vi "Piano PWM AO.vi"() -> ()   [LabVIEW 2024, in "CTI-Scratchpad.lvlib"]
uses:
  CTI/Identity.ctl
  CTI/GPIO Number.ctl
  CTI/Session/Session.lvclass
  CTI-Scratchpad.lvlib
  CTI/VisaComms/VisaComms.lvclass
  CTI/CTI.lvlib
panel:
  out "Identity":T1
  in  "GroveConnector":enum16{"A0", "A1", "A2"}(ring)
  out "error out":errorcluster
  in  "Duty Cycle":dbl(slide)=0.09183673469387754 scale=0.0..1.0
  in  "D5#":bool
  in  "E5":bool
  in  "C5#":bool
  in  "D5":bool
  in  "A4#":bool
  in  "G4#":bool
  in  "F4#":bool
  in  "D4#":bool
  in  "C4#":bool
  in  "VISA resource":refnum<visa-resource-name>="ASRL5::INSTR"
  in  "stop":bool
  in  "C5":bool
  in  "B4":bool
  in  "A4":bool
  in  "G4":bool
  in  "F4":bool
  in  "E4":bool
  in  "D4":bool
  in  "C4":bool
  # "https://wiki.seeedstudio.com/Grove-Passive-Buzzer/"
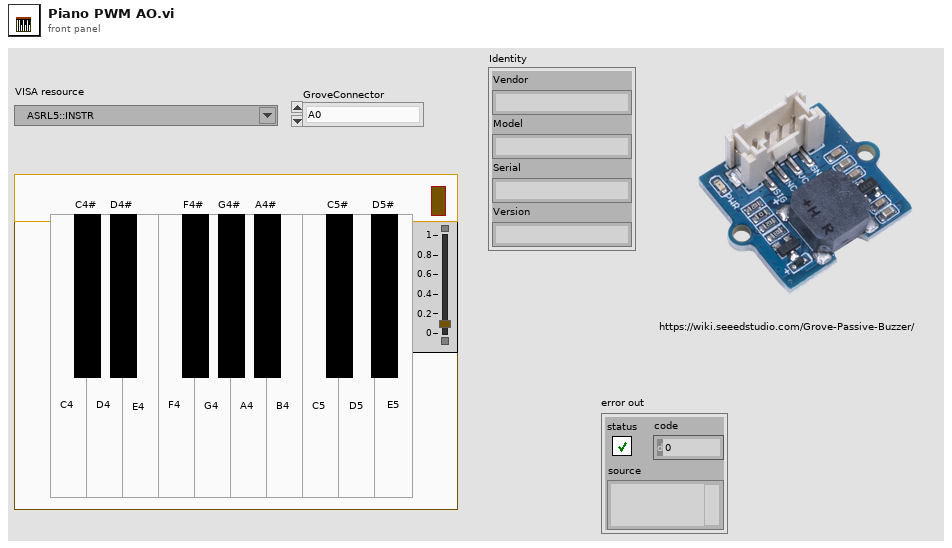
[diagram p1: front panel]
types:
  T1 = typedef "CTI.lvlib/Identity.ctl" = cluster{"Vendor":string, "Model":string, "Serial":string, "Version":string}
  T2 = typedef "CTI.lvlib/GPIO Number.ctl" = i8
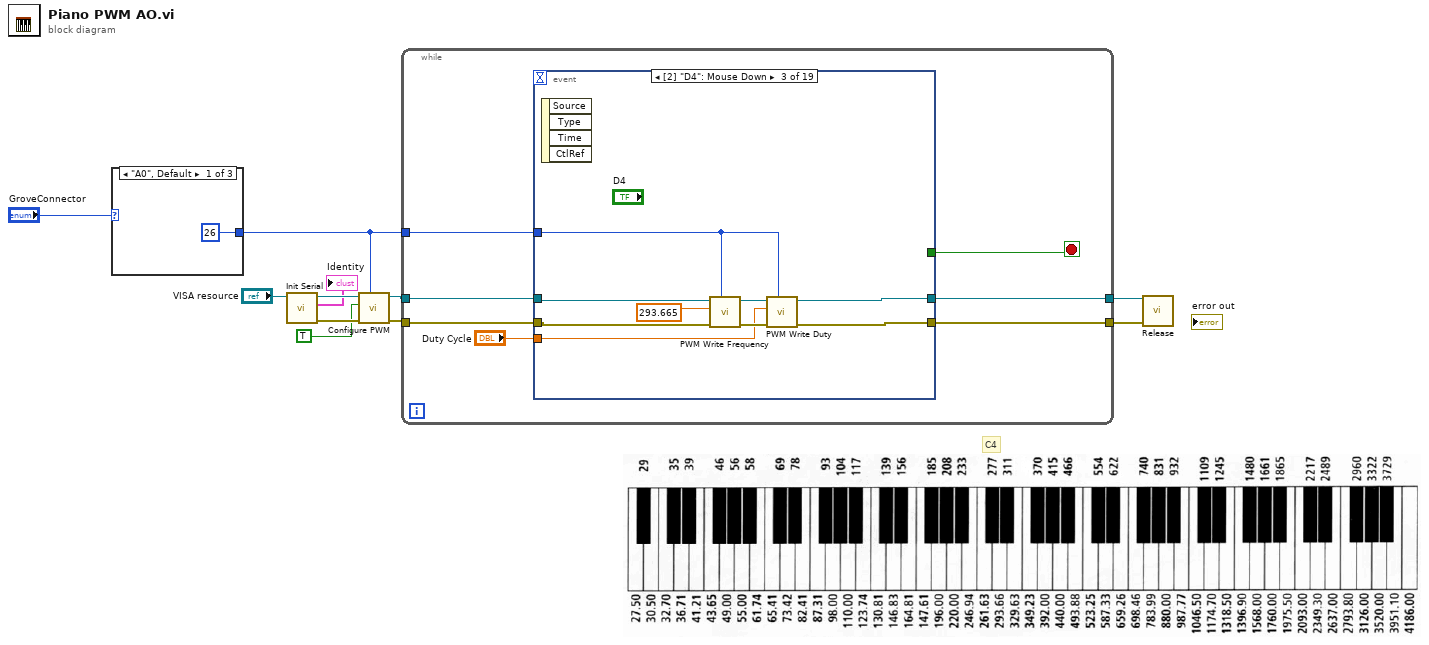
[diagram p0: block diagram]
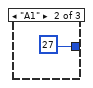
[diagram p2: hidden frame]
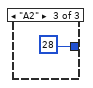
[diagram p3: hidden frame]
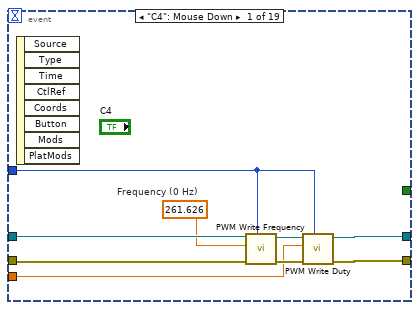
[diagram p4: hidden frame]
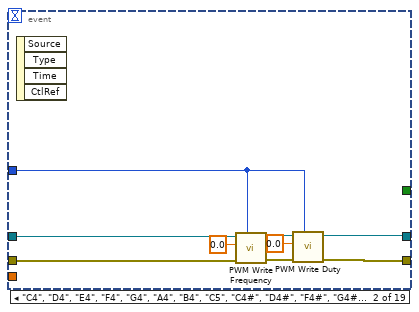
[diagram p5: hidden frame]
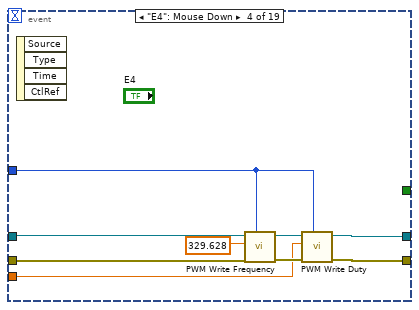
[diagram p6: hidden frame]
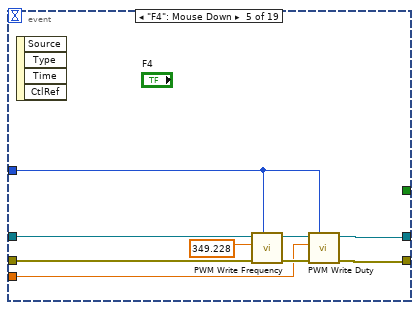
[diagram p7: hidden frame]
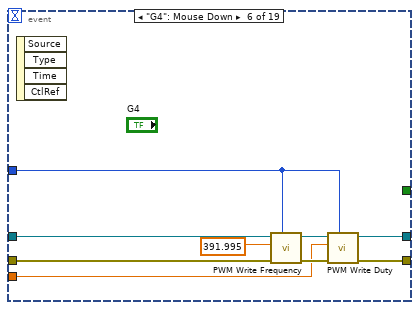
[diagram p8: hidden frame]
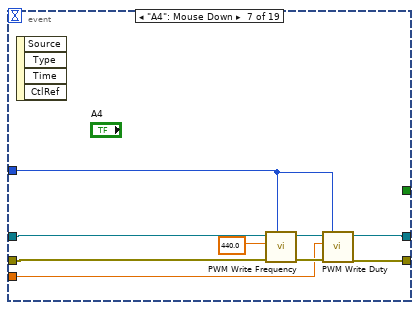
[diagram p9: hidden frame]
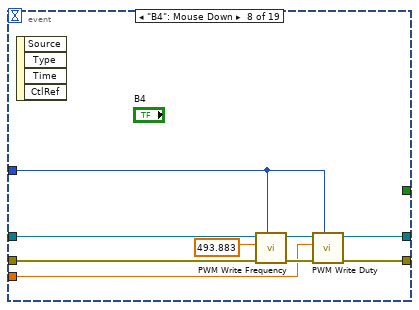
[diagram p10: hidden frame]
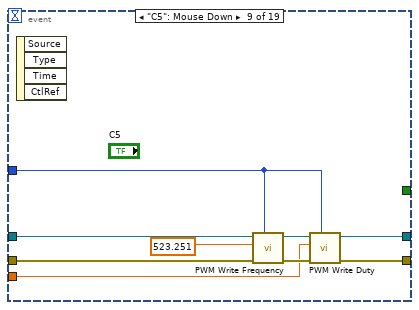
[diagram p11: hidden frame]
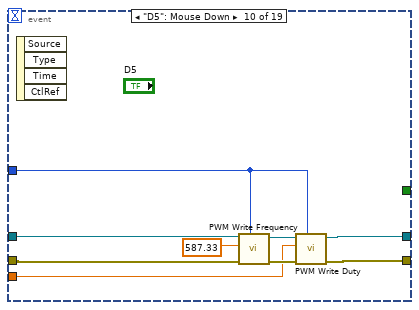
[diagram p12: hidden frame]
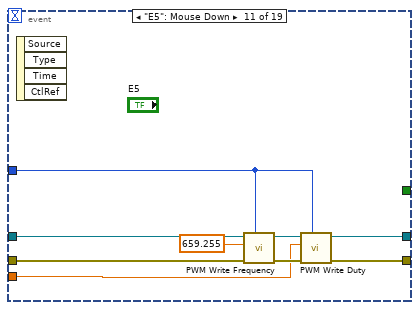
[diagram p13: hidden frame]
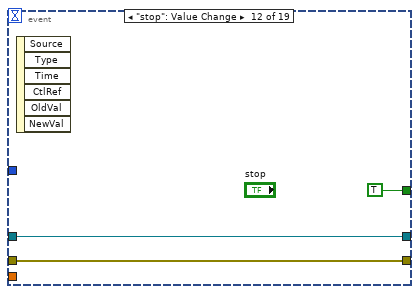
[diagram p14: hidden frame]
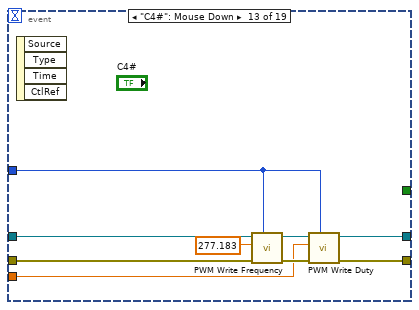
[diagram p15: hidden frame]
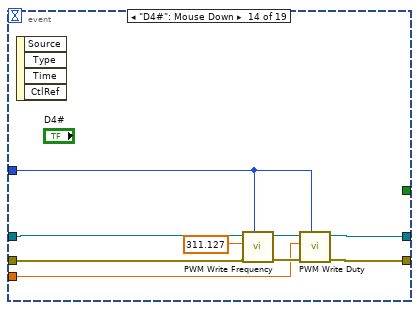
[diagram p16: hidden frame]
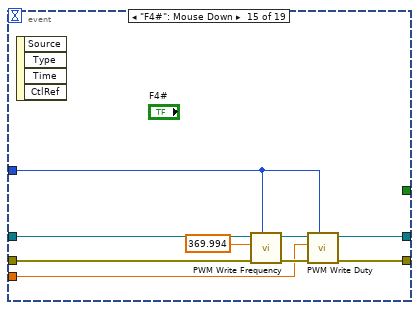
[diagram p17: hidden frame]
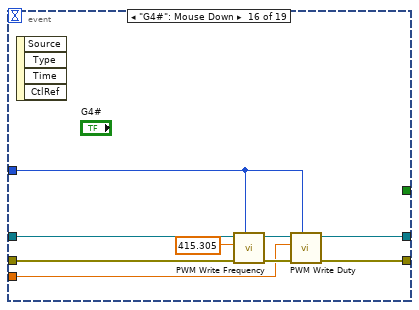
[diagram p18: hidden frame]
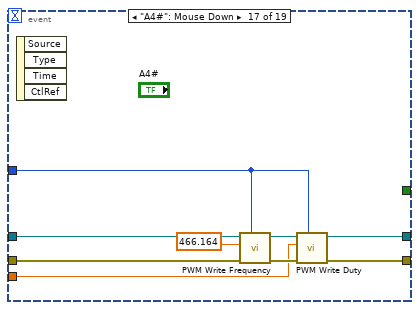
[diagram p19: hidden frame]
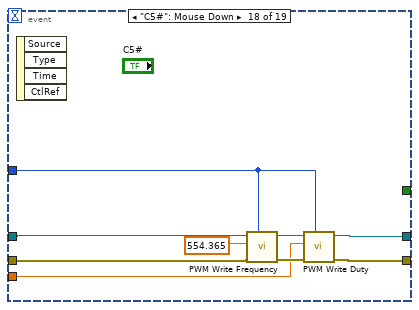
[diagram p20: hidden frame]
diagram:
  # "C4"
  n1 = case shown="\"A0\", Default" "GroveConnector" {
    tunnel: [T2 26 ("GPIO #") T2 27 ("GPIO #") T2 28 ("GPIO #")] -> w3
    frame "A0", Default {
    }
    frame "A1" {
    }
    frame "A2" {
    }
  }
  n2 = call "Init Serial.vi"("VISA resource name in"="VISA resource") -> ("error out"=w9:errorcluster, "Identity"=→"Identity":T1, "Session"=w10:refnum<class "Session.lvclass">)  [unwired: 8 in]
  n3 = call "Configure PWM.vi"("GPIO #"=w3, "error in (no error)"=w9, "Enable (F)"=TRUE, "Session in"=w10) -> ("error out"=w6:errorcluster, "Session out"=w5:refnum<class "Session.lvclass">)  [unwired: 6 in]
  n4 = while {
    tunnel: w5 -> [w20]
    tunnel: w6 -> [w19]
    tunnel: [w16] -> w4
    tunnel: [w17] -> w2
    tunnel: w3 -> [w15]
    stop <- w18 stop-if-true
    n5 = event shown="[2] \"D4\": Mouse Down" {
      selector: _ -> [_ _ _ _ _ _ _ _ _ _ _ _ _ _ _ _ _ _ _]
      dyn-events: _ -> [_ _ _ _ _ _ _ _ _ _ _ _ _ _ _ _ _ _ _]
      timeout: _ -> [_ _ _ _ _ _ _ _ _ _ _ _ _ _ _ _ _ _ _]
      tunnel: "Duty Cycle" -> [w23 _ w44 w53 w61 w69 w80 w85 w95 w103 w113 _ w125 w134 w142 w151 w160 w169 w178]
      tunnel: w20 -> [w25 w37 w47 w55 w64 w71 w78 w90 w97 w106 w116 w122 w127 w136 w145 w155 w163 w173 w181]
      tunnel: w19 -> [w26 w36 w45 w54 w63 w68 w79 w91 w98 w107 w117 w121 w128 w135 w146 w154 w164 w172 w182]
      tunnel: [w27 w35 w41 w49 w59 w72 w81 w87 w94 w108 w118 w121 w129 w138 w147 w156 w165 w174 w183] -> w16
      tunnel: [w28 w34 w42 w50 w60 w73 w82 w88 w100 w109 w114 w122 w130 w139 w148 w157 w166 w175 w184] -> w17
      tunnel: [_ _ _ _ _ _ _ _ _ _ _ TRUE _ _ _ _ _ _ _] -> w18
      tunnel: w15 -> [w22 w33 w40 w51 w58 w67 w76 w89 w99 w104 w115 _ w126 w137 w144 w153 w162 w171 w180]
      event "C4": Mouse Down {
        w24 = 261.626  # Frequency (0 Hz)
        n6 = event-data() -> ()  [unwired: 1 in, 8 out]
        n7 = call "PWM Write Frequency.vi"("GPIO #"=w22, "error in (no error)"=w26, "Frequency Hz"=w24, "Session in"=w25) -> ("error out"=w30:errorcluster, "Session out"=w29:refnum<class "Session.lvclass">)  [unwired: 6 in]
        n8 = call "PWM Write Duty.vi"("GPIO #"=w22, "error in (no error)"=w30, "Duty % (0-1)"=w23, "Session in"=w29) -> ("error out"=w27:errorcluster, "Session out"=w28:refnum<class "Session.lvclass">)  [unwired: 6 in]
      }
      event "C4", "D4", "E4", "F4", "G4", "A4", "B4", "C5", "C4#", "D4#", "F4#", "G4#", "A4#", "C5#", "D5", "D5#", "E5": Mouse Up {
        n9 = event-data() -> ()  [unwired: 1 in, 4 out]
        n10 = call "PWM Write Frequency.vi"("GPIO #"=w33, "error in (no error)"=w36, "Frequency Hz"=sgl 0.0, "Session in"=w37) -> ("error out"=w38:errorcluster, "Session out"=w39:refnum<class "Session.lvclass">)  [unwired: 6 in]
        n11 = call "PWM Write Duty.vi"("GPIO #"=w33, "error in (no error)"=w38, "Duty % (0-1)"=sgl 0.0, "Session in"=w39) -> ("error out"=w35:errorcluster, "Session out"=w34:refnum<class "Session.lvclass">)  [unwired: 6 in]
      }
      event "D4": Mouse Down {
        n12 = event-data() -> ()  [unwired: 1 in, 4 out]
        n13 = call "PWM Write Frequency.vi"("GPIO #"=w40, "error in (no error)"=w45, "Frequency Hz"=293.665 ("Frequency (0 Hz)"), "Session in"=w47) -> ("error out"=w48:errorcluster, "Session out"=w43:refnum<class "Session.lvclass">)  [unwired: 6 in]
        n14 = call "PWM Write Duty.vi"("GPIO #"=w40, "error in (no error)"=w48, "Duty % (0-1)"=w44, "Session in"=w43) -> ("error out"=w41:errorcluster, "Session out"=w42:refnum<class "Session.lvclass">)  [unwired: 6 in]
      }
      event "E4": Mouse Down {
        n15 = event-data() -> ()  [unwired: 1 in, 4 out]
        n16 = call "PWM Write Frequency.vi"("GPIO #"=w51, "error in (no error)"=w54, "Frequency Hz"=329.628 ("Frequency (0 Hz)"), "Session in"=w55) -> ("error out"=w57:errorcluster, "Session out"=w56:refnum<class "Session.lvclass">)  [unwired: 6 in]
        n17 = call "PWM Write Duty.vi"("GPIO #"=w51, "error in (no error)"=w57, "Duty % (0-1)"=w53, "Session in"=w56) -> ("error out"=w49:errorcluster, "Session out"=w50:refnum<class "Session.lvclass">)  [unwired: 6 in]
      }
      event "F4": Mouse Down {
        n18 = event-data() -> ()  [unwired: 1 in, 4 out]
        n19 = call "PWM Write Frequency.vi"("GPIO #"=w58, "error in (no error)"=w63, "Frequency Hz"=349.228, "Session in"=w64) -> ("error out"=w66:errorcluster, "Session out"=w65:refnum<class "Session.lvclass">)  [unwired: 6 in]
        n20 = call "PWM Write Duty.vi"("GPIO #"=w58, "error in (no error)"=w66, "Duty % (0-1)"=w61, "Session in"=w65) -> ("error out"=w59:errorcluster, "Session out"=w60:refnum<class "Session.lvclass">)  [unwired: 6 in]
      }
      event "G4": Mouse Down {
        n21 = event-data() -> ()  [unwired: 1 in, 4 out]
        n22 = call "PWM Write Frequency.vi"("GPIO #"=w67, "error in (no error)"=w68, "Frequency Hz"=391.995, "Session in"=w71) -> ("error out"=w75:errorcluster, "Session out"=w74:refnum<class "Session.lvclass">)  [unwired: 6 in]
        n23 = call "PWM Write Duty.vi"("GPIO #"=w67, "error in (no error)"=w75, "Duty % (0-1)"=w69, "Session in"=w74) -> ("error out"=w72:errorcluster, "Session out"=w73:refnum<class "Session.lvclass">)  [unwired: 6 in]
      }
      event "A4": Mouse Down {
        n24 = event-data() -> ()  [unwired: 1 in, 4 out]
        n25 = call "PWM Write Frequency.vi"("GPIO #"=w76, "error in (no error)"=w79, "Frequency Hz"=440.0, "Session in"=w78) -> ("error out"=w84:errorcluster, "Session out"=w83:refnum<class "Session.lvclass">)  [unwired: 6 in]
        n26 = call "PWM Write Duty.vi"("GPIO #"=w76, "error in (no error)"=w84, "Duty % (0-1)"=w80, "Session in"=w83) -> ("error out"=w81:errorcluster, "Session out"=w82:refnum<class "Session.lvclass">)  [unwired: 6 in]
      }
      event "B4": Mouse Down {
        n27 = event-data() -> ()  [unwired: 1 in, 4 out]
        n28 = call "PWM Write Frequency.vi"("GPIO #"=w89, "error in (no error)"=w91, "Frequency Hz"=493.883, "Session in"=w90) -> ("error out"=w93:errorcluster, "Session out"=w92:refnum<class "Session.lvclass">)  [unwired: 6 in]
        n29 = call "PWM Write Duty.vi"("GPIO #"=w89, "error in (no error)"=w93, "Duty % (0-1)"=w85, "Session in"=w92) -> ("error out"=w87:errorcluster, "Session out"=w88:refnum<class "Session.lvclass">)  [unwired: 6 in]
      }
      event "C5": Mouse Down {
        n30 = event-data() -> ()  [unwired: 1 in, 4 out]
        n31 = call "PWM Write Frequency.vi"("GPIO #"=w99, "error in (no error)"=w98, "Frequency Hz"=523.251, "Session in"=w97) -> ("error out"=w102:errorcluster, "Session out"=w101:refnum<class "Session.lvclass">)  [unwired: 6 in]
        n32 = call "PWM Write Duty.vi"("GPIO #"=w99, "error in (no error)"=w102, "Duty % (0-1)"=w95, "Session in"=w101) -> ("error out"=w94:errorcluster, "Session out"=w100:refnum<class "Session.lvclass">)  [unwired: 6 in]
      }
      event "D5": Mouse Down {
        n33 = event-data() -> ()  [unwired: 1 in, 4 out]
        n34 = call "PWM Write Frequency.vi"("GPIO #"=w104, "error in (no error)"=w107, "Frequency Hz"=587.33, "Session in"=w106) -> ("error out"=w111:errorcluster, "Session out"=w110:refnum<class "Session.lvclass">)  [unwired: 6 in]
        n35 = call "PWM Write Duty.vi"("GPIO #"=w104, "error in (no error)"=w111, "Duty % (0-1)"=w103, "Session in"=w110) -> ("error out"=w108:errorcluster, "Session out"=w109:refnum<class "Session.lvclass">)  [unwired: 6 in]
      }
      event "E5": Mouse Down {
        n36 = event-data() -> ()  [unwired: 1 in, 4 out]
        n37 = call "PWM Write Frequency.vi"("GPIO #"=w115, "error in (no error)"=w117, "Frequency Hz"=659.255, "Session in"=w116) -> ("error out"=w120:errorcluster, "Session out"=w119:refnum<class "Session.lvclass">)  [unwired: 6 in]
        n38 = call "PWM Write Duty.vi"("GPIO #"=w115, "error in (no error)"=w120, "Duty % (0-1)"=w113, "Session in"=w119) -> ("error out"=w118:errorcluster, "Session out"=w114:refnum<class "Session.lvclass">)  [unwired: 6 in]
      }
      event "stop": Value Change {
        n39 = event-data() -> ()  [unwired: 1 in, 6 out]
      }
      event "C4#": Mouse Down {
        n40 = event-data() -> ()  [unwired: 1 in, 4 out]
        n41 = call "PWM Write Frequency.vi"("GPIO #"=w126, "error in (no error)"=w128, "Frequency Hz"=277.183, "Session in"=w127) -> ("error out"=w132:errorcluster, "Session out"=w131:refnum<class "Session.lvclass">)  [unwired: 6 in]
        n42 = call "PWM Write Duty.vi"("GPIO #"=w126, "error in (no error)"=w132, "Duty % (0-1)"=w125, "Session in"=w131) -> ("error out"=w129:errorcluster, "Session out"=w130:refnum<class "Session.lvclass">)  [unwired: 6 in]
      }
      event "D4#": Mouse Down {
        n43 = event-data() -> ()  [unwired: 1 in, 4 out]
        n44 = call "PWM Write Frequency.vi"("GPIO #"=w137, "error in (no error)"=w135, "Frequency Hz"=311.127, "Session in"=w136) -> ("error out"=w141:errorcluster, "Session out"=w140:refnum<class "Session.lvclass">)  [unwired: 6 in]
        n45 = call "PWM Write Duty.vi"("GPIO #"=w137, "error in (no error)"=w141, "Duty % (0-1)"=w134, "Session in"=w140) -> ("error out"=w138:errorcluster, "Session out"=w139:refnum<class "Session.lvclass">)  [unwired: 6 in]
      }
      event "F4#": Mouse Down {
        n46 = event-data() -> ()  [unwired: 1 in, 4 out]
        n47 = call "PWM Write Frequency.vi"("GPIO #"=w144, "error in (no error)"=w146, "Frequency Hz"=369.994, "Session in"=w145) -> ("error out"=w150:errorcluster, "Session out"=w149:refnum<class "Session.lvclass">)  [unwired: 6 in]
        n48 = call "PWM Write Duty.vi"("GPIO #"=w144, "error in (no error)"=w150, "Duty % (0-1)"=w142, "Session in"=w149) -> ("error out"=w147:errorcluster, "Session out"=w148:refnum<class "Session.lvclass">)  [unwired: 6 in]
      }
      event "G4#": Mouse Down {
        n49 = event-data() -> ()  [unwired: 1 in, 4 out]
        n50 = call "PWM Write Frequency.vi"("GPIO #"=w153, "error in (no error)"=w154, "Frequency Hz"=415.305, "Session in"=w155) -> ("error out"=w159:errorcluster, "Session out"=w158:refnum<class "Session.lvclass">)  [unwired: 6 in]
        n51 = call "PWM Write Duty.vi"("GPIO #"=w153, "error in (no error)"=w159, "Duty % (0-1)"=w151, "Session in"=w158) -> ("error out"=w156:errorcluster, "Session out"=w157:refnum<class "Session.lvclass">)  [unwired: 6 in]
      }
      event "A4#": Mouse Down {
        n52 = event-data() -> ()  [unwired: 1 in, 4 out]
        n53 = call "PWM Write Frequency.vi"("GPIO #"=w162, "error in (no error)"=w164, "Frequency Hz"=466.164, "Session in"=w163) -> ("error out"=w168:errorcluster, "Session out"=w167:refnum<class "Session.lvclass">)  [unwired: 6 in]
        n54 = call "PWM Write Duty.vi"("GPIO #"=w162, "error in (no error)"=w168, "Duty % (0-1)"=w160, "Session in"=w167) -> ("error out"=w165:errorcluster, "Session out"=w166:refnum<class "Session.lvclass">)  [unwired: 6 in]
      }
      event "C5#": Mouse Down {
        n55 = event-data() -> ()  [unwired: 1 in, 4 out]
        n56 = call "PWM Write Frequency.vi"("GPIO #"=w171, "error in (no error)"=w172, "Frequency Hz"=554.365, "Session in"=w173) -> ("error out"=w177:errorcluster, "Session out"=w176:refnum<class "Session.lvclass">)  [unwired: 6 in]
        n57 = call "PWM Write Duty.vi"("GPIO #"=w171, "error in (no error)"=w177, "Duty % (0-1)"=w169, "Session in"=w176) -> ("error out"=w174:errorcluster, "Session out"=w175:refnum<class "Session.lvclass">)  [unwired: 6 in]
      }
      event "D5#": Mouse Down {
        n58 = event-data() -> ()  [unwired: 1 in, 8 out]
        n59 = call "PWM Write Frequency.vi"("GPIO #"=w180, "error in (no error)"=w182, "Frequency Hz"=622.254, "Session in"=w181) -> ("error out"=w186:errorcluster, "Session out"=w185:refnum<class "Session.lvclass">)  [unwired: 6 in]
        n60 = call "PWM Write Duty.vi"("GPIO #"=w180, "error in (no error)"=w186, "Duty % (0-1)"=w178, "Session in"=w185) -> ("error out"=w183:errorcluster, "Session out"=w184:refnum<class "Session.lvclass">)  [unwired: 6 in]
      }
    }
  }
  n61 = call-dynamic "Release.vi"("error in (no error)"=w4, "Session in"=w2) -> ()  [unwired: 9 in, 1 out]
